vi "sub_thresh_swing_subvi_07_11a_JW.vi"(0 "Path":path, 5 "Array":string[][](array[string]), 9 "NumPts":dbl=3.0, 11 "Row Start":dbl=20.0) -> (3 "Index":dbl, 4 "XY Graph":cluster{dbl[], dbl[]}[](graph), 12 "Table Control":string[][](table), 13 "Table Control 2":string[][](table), 15 "Sub Threshold Swing":dbl)   [LabVIEW 2011]
uses:
  <vilib>/Utility/file.llb/Read From Spreadsheet File (string).vi
  <vilib>/Analysis/NI_AALPro.lvlib
panel:
  out "Numeric":dbl
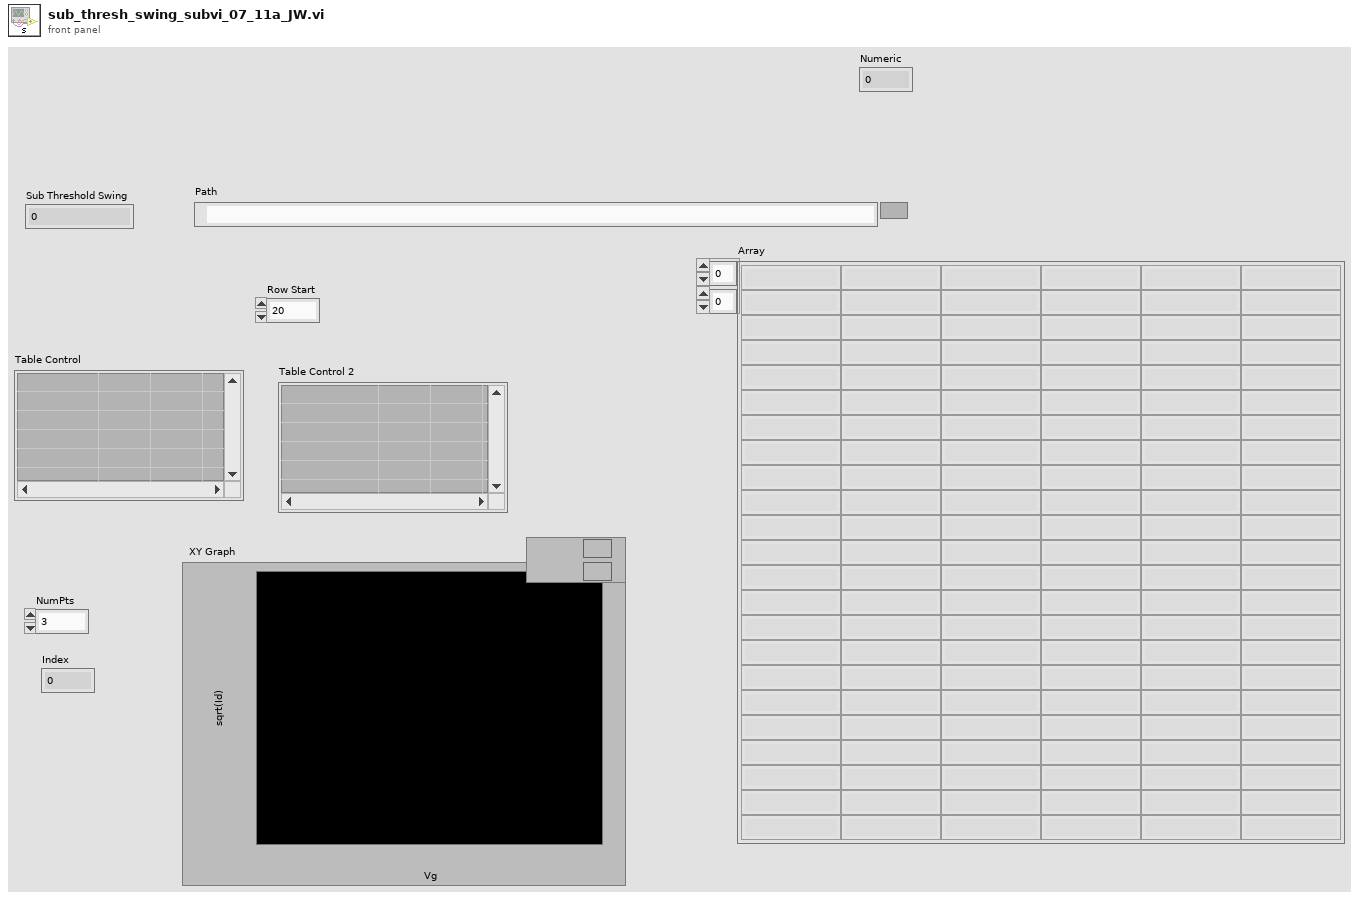
[diagram p1: front panel]
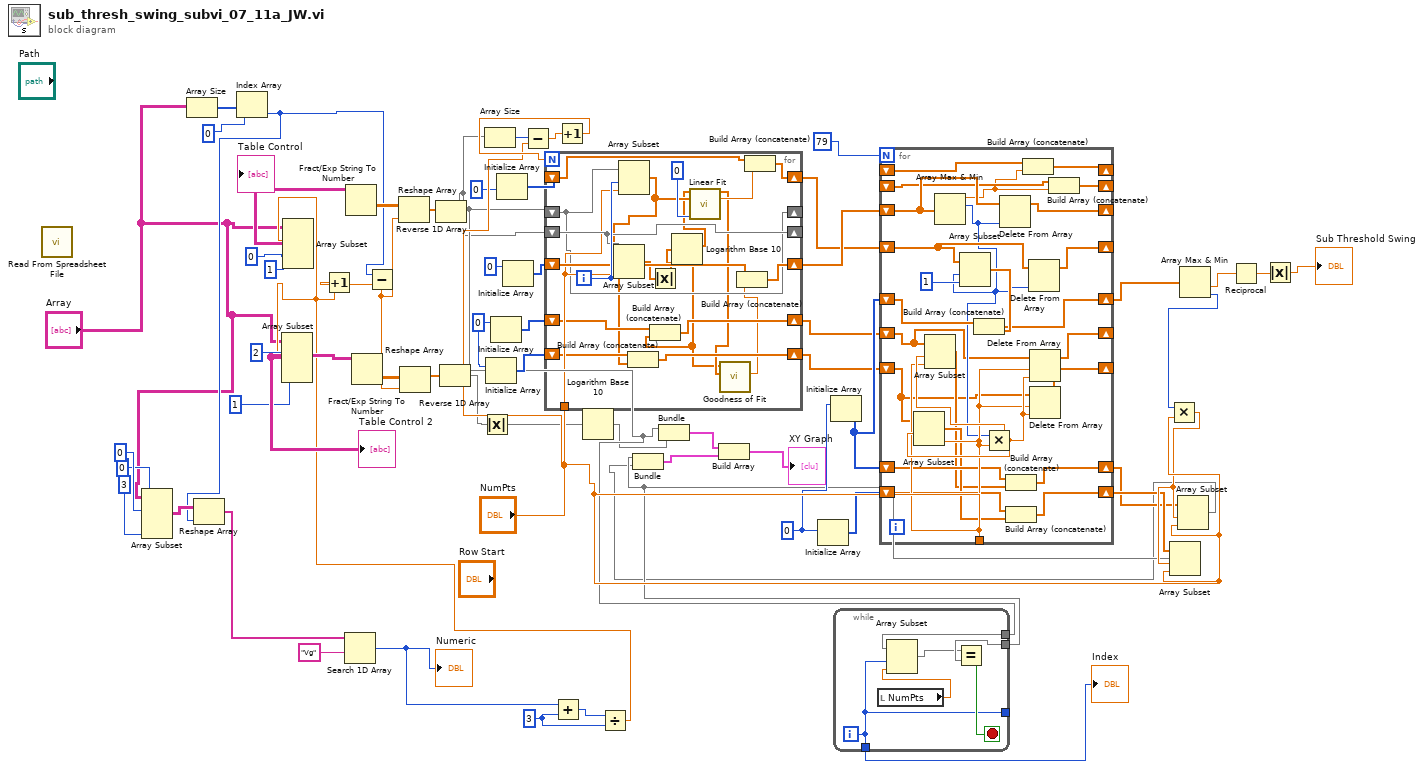
[diagram p0: block diagram]
diagram:
  w12 = 3
  w52 = 0
  w44 = 0
  n1 = call-poly <vilib>:"Read From Spreadsheet File.vi"() -> ()  [unwired: 7 in, 5 out]
  n2 = Array Subset(array="Array", index (row)=0, index (col)=0, length (col)=3) -> (w5:string[][])  [unwired: 1 in]
  n3 = Array Size(array="Array") -> (size(s)=w40:i32[])
  n4 = Index Array(array=w40, index=0) -> (element=w4:i32)
  n5 = Reshape Array(w5, w4) -> (w3:string[])
  n6 = Search 1D Array(1D array=w3, element="Vg") -> (index of element=w10:i32)  [unwired: 1 in]
  "Numeric" <- w10
  n7 = Initialize Array(w44) -> (w46:i32[])  [unwired: 1 in]
  n8 = Initialize Array(w44) -> (w45:i32[])  [unwired: 1 in]
  n9 = Initialize Array(0) -> (w28:i32[])  [unwired: 1 in]
  n10 = Initialize Array(0) -> (w29:i32[])  [unwired: 1 in]
  n11 = Add(x=w10, y=w12) -> (x+y=w11:i32)
  n12 = Divide(x=w11, y=w12) -> (x/y=w2:dbl)
  n13 = Array Subset(array="Array", index (row)=w2, index (col)=2, length (col)=1) -> (w33:string[][])  [unwired: 1 in]
  "Table Control 2" <- w33
  n14 = Array Subset(array="Array", index (row)=w2, index (col)=0, length (col)=1) -> (w32:string[][])  [unwired: 1 in]
  "Table Control" <- w32
  n15 = Increment(x=w2) -> (x+1=w59:dbl)
  n16 = Fract/Exp String To Number(string=w32) -> (number=w34:dbl[][])  [unwired: 3 in, 1 out]
  n17 = Fract/Exp String To Number(string=w33) -> (number=w35:dbl[][])  [unwired: 3 in, 1 out]
  n18 = Subtract(x=w4, y=w59) -> (x-y=w60:dbl)
  n19 = Reshape Array(w34, w60) -> (w49:dbl[])
  n20 = Reshape Array(w35, w60) -> (w50:dbl[])
  n21 = Reverse 1D Array(array=w49) -> (reversed array=w22:dbl[])
  n22 = Reverse 1D Array(array=w50) -> (reversed array=w18:dbl[])
  n23 = Absolute Value(x=w18) -> (abs(x)=w17:dbl[])
  n24 = Array Size(array=w22) -> (size(s)=w27:i32)
  n25 = Subtract(x=w27, y="NumPts") -> (x-y=w62:dbl)
  n26 = Increment(x=w62) -> (x+1=w63:dbl)
  n27 = for {
    N: w63 -> [_]
    shift-right: [w70] -> _
    shift-left: w22 -> [w70]
    shift-right: [w77] -> _
    shift-left: w18 -> [w77]
    shift-right: [w81] -> w37
    shift-left: w28 -> [w80]
    shift-right: [w79] -> w41
    shift-left: w29 -> [w78]
    tunnel: "NumPts" -> [w75]
    shift-right: [w73] -> w47
    shift-left: w45 -> [w74]
    shift-right: [w71] -> w48
    shift-left: w46 -> [w72]
    i -> [w83]
    n28 = Array Subset(array=w77, index=w83, length=w75) -> (w64:dbl[])
    n29 = Array Subset(array=w70, index=w83, length=w75) -> (w69:dbl[])
    n30 = Build Array (concatenate)(w72, w69) -> (w71:dbl[])
    n31 = Absolute Value(x=w64) -> (abs(x)=w65:dbl[])
    n32 = Logarithm Base 10(1:w65) -> (0:w66:dbl[])
    n33 = Build Array (concatenate)(w74, w66) -> (w73:dbl[])
    n34 = call <vilib>:"Linear Fit.vi"("Y"=w66, "X"=w69, "method"=0) -> ("Best Linear Fit"=w68:dbl[], "slope"=w82:dbl)  [unwired: 8 in, 3 out]
    n35 = call <vilib>:"Goodness of Fit.vi"("Best Fit"=w68, "Y"=w66) -> ("R-square"=w67:dbl)  [unwired: 6 in, 3 out]
    n36 = Build Array (concatenate)(w78, w67) -> (w79:dbl[])
    n37 = Build Array (concatenate)(w80, w82) -> (w81:dbl[])
  }
  n38 = Logarithm Base 10(1:w17) -> (0:w19:dbl[])
  n39 = Bundle(w22, w19) -> (w43:cluster{dbl[], dbl[]})  [unwired: 1 in]
  n40 = Initialize Array(w52) -> (w51:i32[])  [unwired: 1 in]
  n41 = Initialize Array(w52) -> (w56:i32[])  [unwired: 1 in]
  n42 = for {
    N: 79 -> [_]
    shift-right: [w108] -> _
    shift-left: w41 -> [w109]
    shift-right: [w88] -> _
    shift-left: w37 -> [w89]
    shift-right: [w105] -> w38
    shift-left: w56 -> [w104]
    shift-right: [w103] -> _
    shift-left: _ -> [w102]
    shift-right: [w101] -> _
    shift-left: _ -> [w100]
    shift-right: [w99] -> _
    shift-left: w47 -> [w85]
    shift-right: [w97] -> _
    shift-left: w48 -> [w84]
    tunnel: "NumPts" -> [w96]
    shift-right: [w95] -> w53
    shift-left: w56 -> [w94]
    shift-right: [w93] -> w54
    shift-left: w51 -> [w92]
    n43 = Array Max & Min(array=w109) -> (max value=w87:dbl, max index (indices)=w86:i32)  [unwired: 2 out]
    n44 = Array Subset(array=w89, index=w86, length=1) -> (w106:dbl[])
    n45 = Build Array (concatenate)(w104, w106) -> (w105:dbl[])
    n46 = Multiply(x=w86, y=w96) -> (x*y=w98:dbl)
    n47 = Array Subset(array=w84, index=w98, length=w96) -> (w91:dbl[])
    n48 = Array Subset(array=w85, index=w98, length=w96) -> (w90:dbl[])
    n49 = Delete From Array(array=w109, index=w86) -> (array with subset deleted=w108:dbl[])  [unwired: 1 in, 1 out]
    n50 = Build Array (concatenate)(w94, w90) -> (w95:dbl[])
    n51 = Build Array (concatenate)(w92, w91) -> (w93:dbl[])
    n52 = Build Array (concatenate)(w102, w87) -> (w103:dbl[])
    n53 = Delete From Array(array=w89, index=w86) -> (array with subset deleted=w88:dbl[])  [unwired: 1 in, 1 out]
    n54 = Delete From Array(array=w85, length=w96, index=w98) -> (array with subset deleted=w99:dbl[])  [unwired: 1 out]
    n55 = Delete From Array(array=w84, length=w96, index=w98) -> (array with subset deleted=w97:dbl[])  [unwired: 1 out]
    n56 = Build Array (concatenate)(w100, w87) -> (w101:dbl[])
  }
  n57 = Array Max & Min(array=w38) -> (min value=w16:dbl, min index (indices)=w55:i32)  [unwired: 2 out]
  n58 = Multiply(x=w55, y="NumPts") -> (x*y=w57:dbl)
  n59 = Array Subset(array=w54, index=w57, length="NumPts") -> (w20:dbl[])
  n60 = while {
    tunnel: [w110] -> _
    tunnel: w22 -> [w114]
    tunnel: w20 -> [w113]
    tunnel: [w110] -> w21
    i -> [w110]
    stop <- w115 stop-if-true
    n61 = local read "NumPts"() -> (w111:dbl)
    n62 = Array Subset(array=w114, index=w110, length=w111) -> (w112:dbl[])
    n63 = Equal?(x=w112, y=w113) -> (x = y?=w115:bool)
  }
  "Index" <- w21
  n64 = Array Subset(array=w53, index=w57, length="NumPts") -> (w13:dbl[])
  n65 = Bundle(w20, w13) -> (w58:cluster{dbl[], dbl[]})  [unwired: 1 in]
  n66 = Build Array(w43, w58) -> (→"XY Graph":cluster{dbl[], dbl[]}[])
  n67 = Reciprocal(x=w16) -> (1/x=w15:dbl)
  n68 = Absolute Value(x=w15) -> (abs(x)=→"Sub Threshold Swing":dbl)
